vi "Chrg_Dschrg.vi"(3 "Strain Offset":dbl, 4 "PS VISA in":refnum<visa-resource-name>, 5 "PS error in":errorcluster caption="PS error in (no error)", 6 "CyclePath":path=path "C:/Users/ga11/Desktop/VI/results/3PtestCharge.lvm" caption="Filename", 7 "Battery Type":T1(ring), 8 "Charge/discharge":enum8{"Charge", "Discharge"}(ring), 9 "Charge/Discharge Voltage Setpoint":dbl format="%#.6g", 11 "Current Setpoint":dbl format="%#.6g", 13 "Current Cutoff":dbl) -> (14 "PS VISA out":refnum<visa-resource-name>, 16 "Boolean":bool, 19 "PS error out":errorcluster)   [LabVIEW 2020]
uses:
  <vilib>/Utility/TradDaqScaling.llb/Convert Strain Gauge Reading (scaler).vi
  Drivers-IT-M3400/IT-M3400.lvlib
panel:
  out "Read Current(A)":dbl format="%.2g"
  out "Read Voltage(V)":dbl format="%.2g"
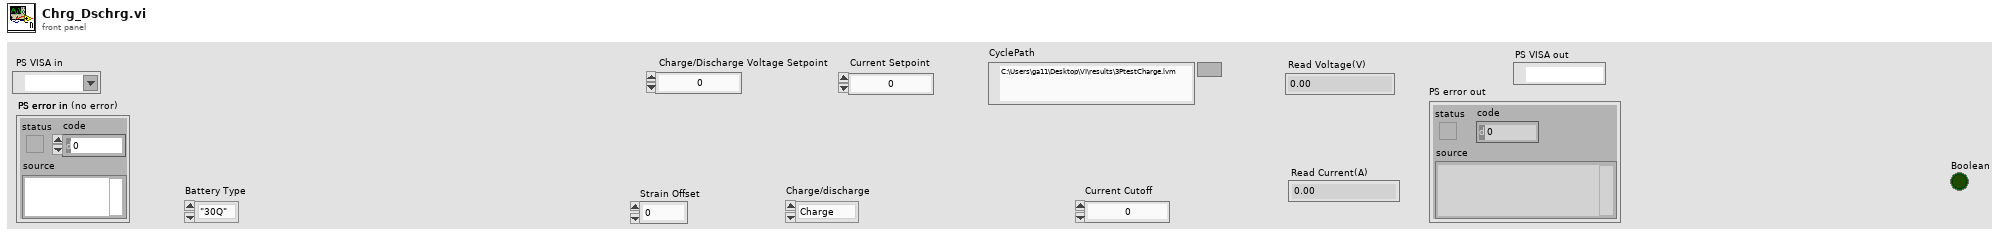
[diagram p1: front panel]
types:
  T1 = enum16{"\"30Q\"", "\"40T\"", "\"2P30Q\"", "\"3P30Q\"", "\"Nissan Leaf\""}
  T2 = cluster{"Baud Rate":u32, "Parity":u16, "Data Bits":u16, "Stop Bits":u16, "Flow Control":u16}
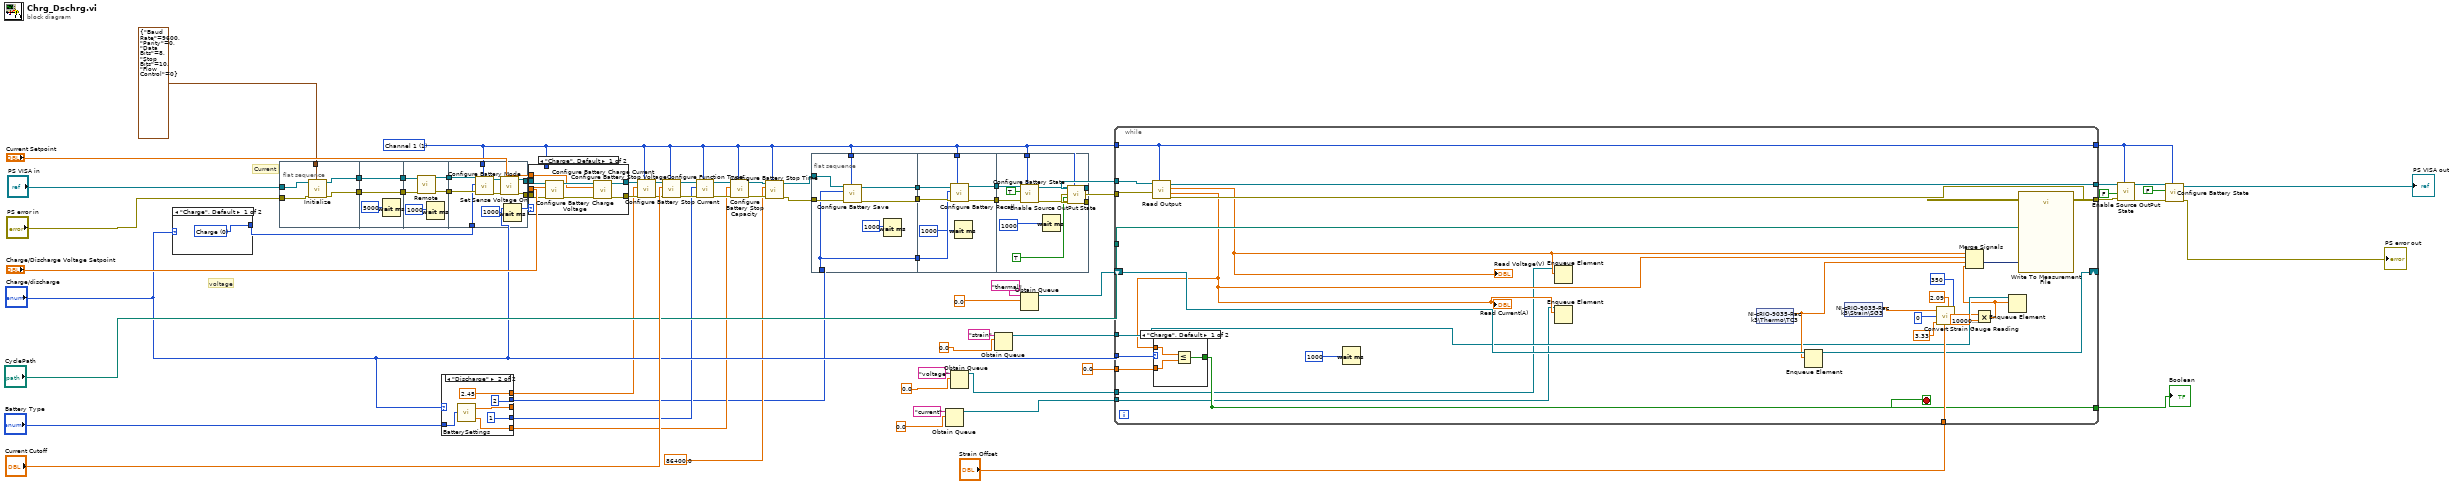
[diagram p0: block diagram]
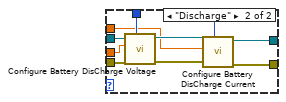
[diagram p2: hidden frame]
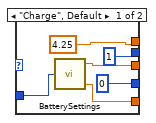
[diagram p3: hidden frame]
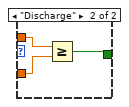
[diagram p4: hidden frame]
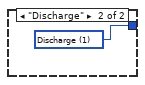
[diagram p5: hidden frame]
diagram:
  w19 = 1 items=["Channel 1"=1, "Channel 2"=2, "Channel 3"=3, "Channel 4"=4, "Channel 5"=5, "Channel 6"=6, "Channel 7"=7, "Channel 8"=8, "Channel 8"=9, "Channel 10"=10, "Channel 11"=11, "Channel 12"=12, "Channel 13"=13, "Channel 14"=14, "Channel 15"=15, "Channel 16"=16] ("Channel")
  # "voltage"
  # "Current"
  n1 = case shown="\"Charge\", Default" "Charge/discharge" {
    tunnel: [w68 w69] -> w27
    frame "Charge", Default {
      w68 = u8 0 items=["Charge", "Discharge"] ("Battery Mode")
    }
    frame "Discharge" {
      w69 = u8 1 items=["Charge", "Discharge"] ("Battery Mode")
    }
  }
  n2 = flat-sequence {
    tunnel: [w70] -> w52
    tunnel: [w71] -> w51
    tunnel: T2 {"Baud Rate"=9600, "Parity"=0, "Data Bits"=8, "Stop Bits"=10, "Flow Control"=0} ("Serial Configuration") -> [w74]
    tunnel: "PS error in" -> [w73]
    tunnel: "PS VISA in" -> [w72]
    tunnel: w52 -> [w77]
    tunnel: [w77] -> w50
    tunnel: w51 -> [w76]
    tunnel: [w76] -> w49
    tunnel: [w82] -> w48
    tunnel: [w81] -> w47
    tunnel: w50 -> [w80]
    tunnel: w49 -> [w79]
    tunnel: w48 -> [w88]
    tunnel: w47 -> [w90]
    tunnel: w19 -> [w91]
    tunnel: w27 -> [w89]
    tunnel: [w83] -> w16
    tunnel: [w84] -> w15
    frame #0 {
      n3 = call "Initialize.vi"("Serial Configuration"=w74, "error in"=w73, "VISA resource name"=w72) -> ("error out"=w71:errorcluster, "VISA resource name out"=w70:refnum<visa-resource-name>)  [unwired: 7 in]
    }
    frame #1 {
      n4 = Wait (ms)(milliseconds to wait=5000) -> ()  [unwired: 1 out]
    }
    frame #2 {
      n5 = call "Remote.vi"("error in"=w79, "VISA resource name"=w80) -> ("error out"=w81:errorcluster, "VISA resource name out"=w82:refnum<visa-resource-name>)  [unwired: 8 in]
      n6 = Wait (ms)(milliseconds to wait=1000) -> ()  [unwired: 1 out]
    }
    frame #3 {
      n7 = call "Configure Battery Mode.vi"("Channel"=w91, "error in"=w90, "Battery Mode"=w89, "VISA resource name"=w88) -> ("error out"=w85:errorcluster, "VISA resource name out"=w86:refnum<visa-resource-name>)  [unwired: 6 in]
      n8 = call "Set Sense Voltage On.vi"("error in"=w85, "VISA resource name"=w86) -> ("error out"=w83:errorcluster, "VISA resource name out"=w84:refnum<visa-resource-name>)  [unwired: 8 in]
      n9 = Wait (ms)(milliseconds to wait=1000) -> ()  [unwired: 1 out]
    }
  }
  n10 = case shown="\"Discharge\"" "Charge/discharge" {
    tunnel: "Battery Type" -> [w97 w103]
    tunnel: [w96 w101] -> _
    tunnel: [u8 0 ("File") u8 1 ("File")] -> w21
    tunnel: [u8 1 ("File") u8 2 ("File")] -> w18
    tunnel: [w93 w99] -> w20
    tunnel: [4.25 2.45] -> w17
    frame "Charge", Default {
      n11 = call "BatterySettings.vi"("Battery Type"=w97) -> ("RatedCapacity (Ah)"=w93:dbl, "Max Voltage (V)"=w96:dbl)  [unwired: 2 in, 1 out]
    }
    frame "Discharge" {
      n12 = call "BatterySettings.vi"("Battery Type"=w103) -> ("RatedCapacity (Ah)"=w99:dbl, "Min Voltage (V)"=w101:dbl)  [unwired: 2 in, 1 out]
    }
  }
  n13 = case shown="\"Charge\", Default" "Charge/discharge" {
    tunnel: w15 -> [w111 w120]
    tunnel: w16 -> [w110 w119]
    tunnel: [w105 w116] -> w38
    tunnel: [w104 w115] -> w37
    tunnel: w19 -> [_ w114]
    tunnel: "Charge/Discharge Voltage Setpoint" -> [w107 w113]
    tunnel: "Current Setpoint" -> [w106 w112]
    frame "Charge", Default {
      n14 = call "Configure Battery Charge Voltage.vi"("error in"=w110, "Charge Voltage(V)"=w107, "VISA resource name"=w111) -> ("error out"=w108:errorcluster, "VISA resource name out"=w109:refnum<visa-resource-name>)  [unwired: 6 in]
      n15 = call "Configure Battery Charge Current.vi"("error in"=w108, "Charge Current(A)"=w106, "VISA resource name"=w109) -> ("error out"=w104:errorcluster, "VISA resource name out"=w105:refnum<visa-resource-name>)  [unwired: 7 in]
    }
    frame "Discharge" {
      n16 = call "Configure Battery DisCharge Voltage.vi"("Channel"=w114, "error in"=w119, "Discharge Voltage(V)"=w113, "VISA resource name"=w120) -> ("error out"=w117:errorcluster, "VISA resource name out"=w118:refnum<visa-resource-name>)  [unwired: 6 in]
      n17 = call "Configure Battery DisCharge Current.vi"("Channel"=w114, "error in"=w117, "Discharge Current(A)"=w112, "VISA resource name"=w118) -> ("error out"=w115:errorcluster, "VISA resource name out"=w116:refnum<visa-resource-name>)  [unwired: 6 in]
    }
  }
  n18 = call "Configure Battery Stop Voltage.vi"("Channel"=w19, "error in"=w37, "Stop Voltage(V)"=w17, "VISA resource name"=w38) -> ("error out"=w45:errorcluster, "VISA resource name out"=w46:refnum<visa-resource-name>)  [unwired: 6 in]
  n19 = call "Configure Battery Stop Current.vi"("Channel"=w19, "error in"=w45, "Stop Current(A)"="Current Cutoff", "VISA resource name"=w46) -> ("error out"=w23:errorcluster, "VISA resource name out"=w25:refnum<visa-resource-name>)  [unwired: 6 in]
  n20 = call "Configure Function Type.vi"("Channel"=w19, "error in"=w23, "Function Type"=w21, "VISA resource name"=w25) -> ("error out"=w22:errorcluster, "VISA resource name out"=w24:refnum<visa-resource-name>)  [unwired: 6 in]
  n21 = call "Configure Battery Stop Capacity.vi"("Channel"=w19, "error in"=w22, "Stop Capacity(Ah)"=w20, "VISA resource name"=w24) -> ("error out"=w43:errorcluster, "VISA resource name out"=w44:refnum<visa-resource-name>)  [unwired: 6 in]
  n22 = call "Configure Battery Stop Time.vi"("Channel"=w19, "error in"=w43, "Stop Time(S)"=86400.0, "VISA resource name"=w44) -> ("error out"=w29:errorcluster, "VISA resource name out"=w28:refnum<visa-resource-name>)  [unwired: 6 in]
  n23 = flat-sequence {
    tunnel: w18 -> [w126]
    tunnel: w19 -> [w121]
    tunnel: [w124] -> w57
    tunnel: [w126] -> w56
    tunnel: [w123] -> w55
    tunnel: w29 -> [w127]
    tunnel: w28 -> [w125]
    tunnel: [w130] -> w54
    tunnel: [w131] -> w53
    tunnel: w57 -> [w134]
    tunnel: w56 -> [w133]
    tunnel: w55 -> [w132]
    tunnel: w19 -> [w128]
    tunnel: [w138] -> w36
    tunnel: [w137] -> w35
    tunnel: w19 -> [w136]
    tunnel: w54 -> [w144]
    tunnel: w53 -> [w143]
    frame #0 {
      n24 = call "Configure Battery Save.vi"("Channel"=w121, "error in"=w127, "File"=w126, "VISA resource name"=w125) -> ("error out"=w124:errorcluster, "VISA resource name out"=w123:refnum<visa-resource-name>)  [unwired: 6 in]
      n25 = Wait (ms)(milliseconds to wait=1000) -> ()  [unwired: 1 out]
    }
    frame #1 {
      n26 = call "Configure Battery Recall.vi"("Channel"=w128, "error in"=w134, "File"=w133, "VISA resource name"=w132) -> ("error out"=w131:errorcluster, "VISA resource name out"=w130:refnum<visa-resource-name>)  [unwired: 6 in]
      n27 = Wait (ms)(milliseconds to wait=1000) -> ()  [unwired: 1 out]
    }
    frame #2 {
      n28 = call "Configure Battery State.vi"("Channel"=w136, "error in"=w143, "State"=TRUE, "VISA resource name"=w144) -> ("error out"=w141:errorcluster, "VISA resource name out"=w142:refnum<visa-resource-name>)  [unwired: 6 in]
      n29 = Wait (ms)(milliseconds to wait=1000) -> ()  [unwired: 1 out]
      n30 = call "Enable Source OutPut State.vi"("Channel"=w136, "error in"=w141, "State"=TRUE ("Enable Output|Intput"), "VISA resource name"=w142) -> ("error out"=w137:errorcluster, "VISA resource name out"=w138:refnum<visa-resource-name>)  [unwired: 6 in]
    }
  }
  n31 = Obtain Queue(name (unnamed)="current", element data type=0.0) -> (queue out=w5:refnum<queue>)  [unwired: 3 in, 2 out]
  n32 = Obtain Queue(name (unnamed)="voltage", element data type=0.0) -> (queue out=w6:refnum<queue>)  [unwired: 3 in, 2 out]
  n33 = Obtain Queue(name (unnamed)="strain", element data type=0.0) -> (queue out=w9:refnum<queue>)  [unwired: 3 in, 2 out]
  n34 = Obtain Queue(name (unnamed)="thermal", element data type=0.0) -> (queue out=w12:refnum<queue>)  [unwired: 3 in, 2 out]
  n35 = while {
    tunnel: [w165] -> w34
    tunnel: [w163] -> w33
    tunnel: w36 -> [w172]
    tunnel: w35 -> [w171]
    tunnel: w19 -> [w164]
    tunnel: [w164] -> w32
    tunnel: "CyclePath" -> [w169]
    tunnel: 0.0 -> [w167]
    tunnel: "Charge/discharge" -> [w166]
    tunnel: "Strain Offset" -> [w158]
    shift-right: [w154] -> _
    shift-left: w12 -> [w157]
    tunnel: [w155] -> w11
    tunnel: w9 -> [w153]
    tunnel: w6 -> [w146]
    tunnel: w5 -> [w145]
    stop <- w155 stop-if-true
    n36 = call "Read Output.vi"("Channel"=w164, "error in"=w171, "VISA resource name"=w172) -> ("error out"=w163:errorcluster, "Read Current(A)"=w147:dbl, "Read Voltage(V)"=w148:dbl, "VISA resource name out"=w165:refnum<visa-resource-name>)  [unwired: 5 in]
    "Read Voltage(V)" <- w148
    "Read Current(A)" <- w147
    n37 = case shown="\"Charge\", Default" w166 {
      tunnel: w167 -> [w174 w177]
      tunnel: w147 -> [w175 w178]
      tunnel: [w173 w176] -> w155
      frame "Charge", Default {
        n38 = Less Or Equal?(x=w175, y=w174) -> (x <= y?=w173:bool)
      }
      frame "Discharge" {
        n39 = Greater Or Equal?(x=w178, y=w177) -> (x >= y?=w176:bool)
      }
    }
    n40 = Wait (ms)(milliseconds to wait=1000) -> ()  [unwired: 1 out]
    n41 = Enqueue Element(queue=w145, element=w147) -> ()  [unwired: 2 in, 3 out]
    n42 = Enqueue Element(queue=w146, element=w148) -> ()  [unwired: 2 in, 3 out]
    n43 = shared-variable "NI-cRIO-9035-Rack3\\Thermo\\TC3"() -> (w156:dbl)  [unwired: 1 in, 1 out]
    n44 = Enqueue Element(queue=w157, element=w156) -> (queue out=w154:refnum<queue>)  [unwired: 2 in, 2 out]
    n45 = shared-variable "NI-cRIO-9035-Rack3\\Strain\\SG3"() -> (w152:dbl)  [unwired: 1 in, 1 out]
    n46 = call-poly <vilib>:"Convert Strain Gauge Reading.vi"("Vsg (0.0)"=w152, "Bridge Configuration\n(3:Half Bridge II)"=0, "Vex (3.33)"=3.33, "Vinit (0.0)"=w158, "GF (2.0)"=2.09, "Rg (120)"=350) -> ("Strain"=w151:sgl)  [unwired: 4 in]
    n47 = Multiply(x=w151, y=sgl 1000000.0) -> (x*y=w149:sgl)
    n48 = Merge Signals "Merge Signals"(w148, w147, w156, w149) -> (w170:dynamicdata)
    n49 = Enqueue Element(queue=w153, element=w149) -> ()  [unwired: 2 in, 3 out]
    n50 = call "Write To Measurement File"("Signals"=w170, "Filename"=w169) -> ()  [unwired: 15 in, 3 out]
  }
  "Boolean" <- w11
  n51 = call "Enable Source OutPut State.vi"("Channel"=w32, "error in"=w33, "State"=FALSE, "VISA resource name"=w34) -> ("error out"=w41:errorcluster, "VISA resource name out"=w42:refnum<visa-resource-name>)  [unwired: 6 in]
  n52 = call "Configure Battery State.vi"("Channel"=w32, "error in"=w41, "State"=FALSE, "VISA resource name"=w42) -> ("error out"=→"PS error out":errorcluster, "VISA resource name out"=→"PS VISA out":refnum<visa-resource-name>)  [unwired: 6 in]
